vi "Stop.vi"(8 "error in (no error)":errorcluster, 11 "AODAcq in":refnum<class "AODAcq.lvclass">) -> (0 "error out":errorcluster, 3 "AODAcq out":refnum<class "AODAcq.lvclass">)   [LabVIEW 2011, in "AODAcq.lvclass"]
uses:
  AODAcq.lvclass
  <vilib>/rvi/interface/RandomDataEmulation/nirviRandomDataDMAMethods.vi
  <vilib>/rvi/interface/nirviMethod/nirviMethod.xnode
  FPGA_Control/AODRef.ctl
  FPGA_Control/AOD Control (FPGA).vi
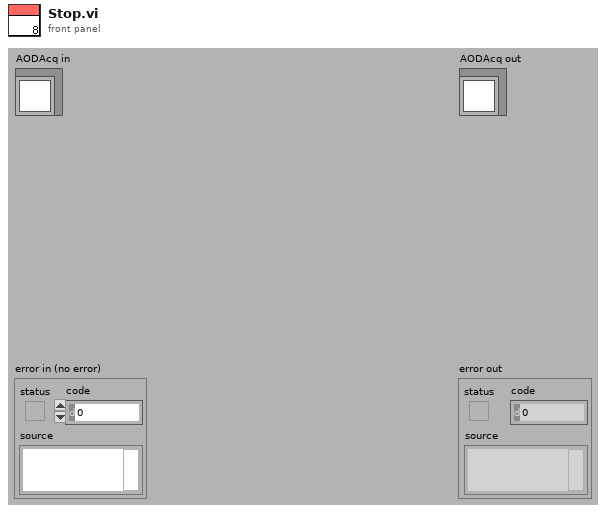
[diagram p1: front panel]
types:
  T1 = cluster{"file handle out":u32, "ImData":u32[], "TemporalData":u32[], "MotionData":u32[], "stream reference":u32, "Open":bool, "RecordRaw":bool}
  T2 = typedef "AODRef.ctl" = refnum<k20>
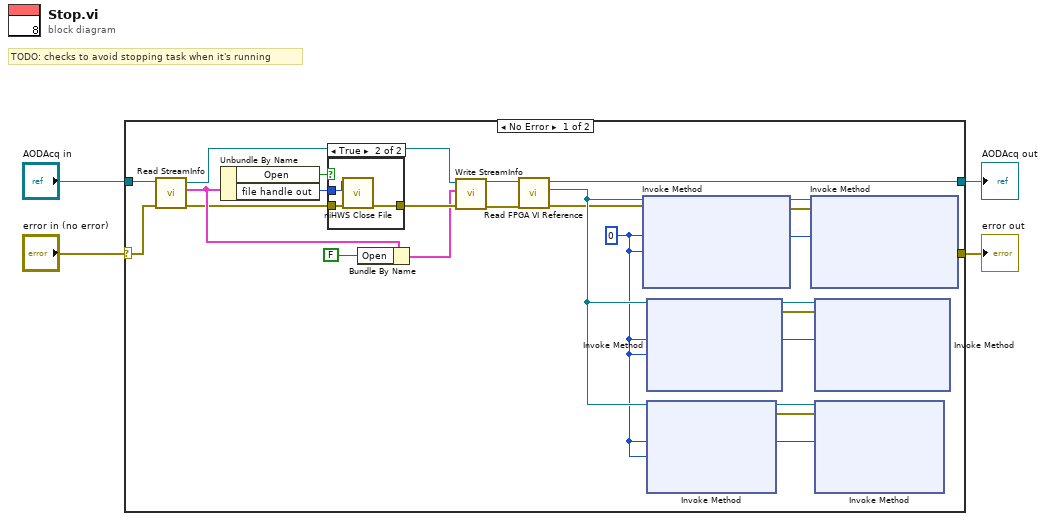
[diagram p0: block diagram]
diagram:
  # "TODO: checks to avoid stopping task when it's running"
  n1 = case shown="No Error" "error in (no error)" {
    selector: "error in (no error)" -> [w5 w36]
    tunnel: [w7 w36] -> w3
    tunnel: [w9 w35] -> w1
    tunnel: "AODAcq in" -> [w6 w35]
    frame No Error {
      w13 = u32 0 ("Number of Elements")
      n2 = call-dynamic "Read StreamInfo.vi"("error in (no error)"=w5, "AODAcq in"=w6) -> ("error out"=w27:errorcluster, "StreamInfo"=w29:T1, "AODAcq out"=w24:refnum<class "AODAcq.lvclass">)  [unwired: 7 in]
      n3 = Unbundle By Name(w29) -> ("Open"=w23:bool, "file handle out"=w30:u32)
      n4 = case shown="True" w23 {
        tunnel: w30 -> [_ w34]
        tunnel: w27 -> [w31 w33]
        tunnel: [w31 w32] -> w26
        frame False {
        }
        frame True {
          n5 = call <instrlib>:"niHWS Close File.vi"("error in (no error)"=w33, "file handle"=w34) -> ("error out"=w32:errorcluster)  [unwired: 9 in]
        }
      }
      n6 = Bundle By Name(cluster=w29, "Open"=FALSE) -> (w25:T1)
      n7 = call-dynamic "Write StreamInfo.vi"("error in (no error)"=w26, "StreamInfo"=w25, "AODAcq in"=w24) -> ("error out"=w22:errorcluster, "AODAcq out"=w21:refnum<class "AODAcq.lvclass">)  [unwired: 7 in]
      n8 = call-dynamic "Read FPGA VI Reference.vi"("error in (no error)"=w22, "AODAcq in"=w21) -> ("error out"=w8:errorcluster, "FPGA VI Reference"=w20:T2, "AODAcq out"=w9:refnum<class "AODAcq.lvclass">)  [unwired: 7 in]
      n9 = xnode "Invoke Method"("FPGA VI Reference In"=w20, "error in"=w8, "Number of Elements"=w13, "Timeout (ms)"=w13) -> ("FPGA VI Reference Out"=w19:T2, "error out"=w18:errorcluster, "Elements Remaining"=w10:u32)  [unwired: 1 out]
      n10 = xnode "Invoke Method"("FPGA VI Reference In"=w20, "Number of Elements"=w13, "Timeout (ms)"=w13) -> ("FPGA VI Reference Out"=w17:T2, "error out"=w16:errorcluster, "Elements Remaining"=w11:u32)  [unwired: 1 in, 1 out]
      n11 = xnode "Invoke Method"("FPGA VI Reference In"=w20, "Number of Elements"=w13, "Timeout (ms)"=w13) -> ("FPGA VI Reference Out"=w15:T2, "error out"=w14:errorcluster, "Elements Remaining"=w12:u32)  [unwired: 1 in, 1 out]
      n12 = xnode "Invoke Method"("FPGA VI Reference In"=w19, "error in"=w18, "Number of Elements"=w10) -> ("error out"=w7:errorcluster)  [unwired: 1 in, 3 out]
      n13 = xnode "Invoke Method"("FPGA VI Reference In"=w17, "error in"=w16, "Number of Elements"=w11) -> ()  [unwired: 1 in, 4 out]
      n14 = xnode "Invoke Method"("FPGA VI Reference In"=w15, "error in"=w14, "Number of Elements"=w12) -> ()  [unwired: 1 in, 4 out]
    }
    frame Error {
    }
  }
  "error out" <- w3
  "AODAcq out" <- w1
